vi "MeasurementServer_Start.vi"(7 "error in (no error)":errorcluster, 8 "Server Key File (.key)":path, 9 "Server Certificate File (.crt)":path, 10 "Server Address":string) -> (0 "error out":errorcluster, 2 "Event Registration Refnum":refnum<event-registration>, 3 "Server Information":T2)   [LabVIEW 2019, in "labview-grpc-measurement-server.lvlib"]
uses:
  labview-grpc-measurement-server.lvlib
  MeasurementServer_InvokeEventData.ctl
  MeasurementServer_gRPCid.ctl
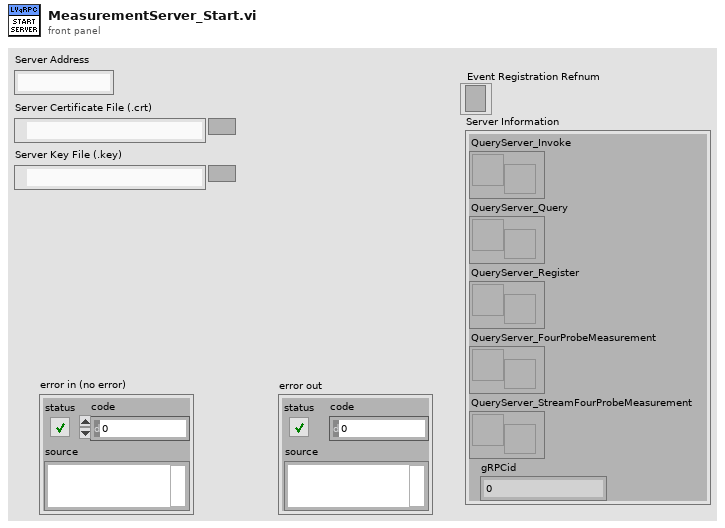
[diagram p1: front panel]
types:
  T1 = typedef "labview-grpc-measurement-server.lvlib/MeasurementServer_gRPCid.ctl" = u64
  T2 = cluster{"QueryServer_Invoke":refnum<user-event>, "QueryServer_Query":refnum<user-event>, "QueryServer_Register":refnum<user-event>, "QueryServer_FourProbeMeasurement":refnum<user-event>, "QueryServer_StreamFourProbeMeasurement":refnum<user-event>, "gRPCid":T1}
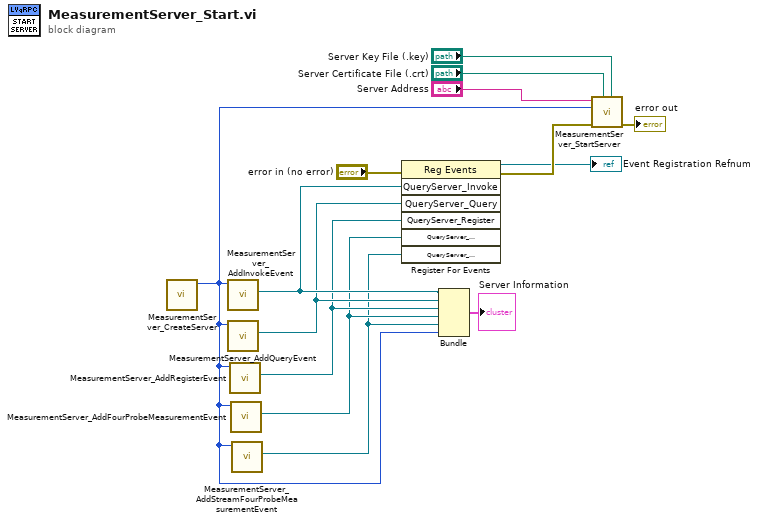
[diagram p0: block diagram]
diagram:
  n1 = call "MeasurementServer_CreateServer.vi"() -> ("gRPCid"=w4:T1)  [unwired: 11 in]
  n2 = call "MeasurementServer_AddInvokeEvent.vi"("gRPCid in"=w4) -> ("QueryServer_Invoke"=w9:refnum<user-event>)  [unwired: 9 in, 1 out]
  n3 = call "MeasurementServer_AddQueryEvent.vi"("gRPCid in"=w4) -> ("QueryServer_Query"=w8:refnum<user-event>)  [unwired: 9 in, 1 out]
  n4 = call "MeasurementServer_AddRegisterEvent.vi"("gRPCid in"=w4) -> ("QueryServer_Register"=w7:refnum<user-event>)  [unwired: 9 in, 1 out]
  n5 = call "MeasurementServer_AddFourProbeMeasurementEvent.vi"("gRPCid in"=w4) -> ("QueryServer_FourProbeMeasurement"=w6:refnum<user-event>)  [unwired: 9 in, 1 out]
  n6 = call "MeasurementServer_AddStreamFourProbeMeasurementEvent.vi"("gRPCid in"=w4) -> ("QueryServer_StreamFourProbeMeasurement"=w5:refnum<user-event>)  [unwired: 9 in, 1 out]
  n7 = register-events(error in="error in (no error)", w9, w8, w7, w6, w5) -> (reference out=→"Event Registration Refnum":refnum<event-registration>, error out=w10:errorcluster)  [unwired: 1 in]
  n8 = Bundle("QueryServer_Invoke"=w9, "QueryServer_Query"=w8, "QueryServer_Register"=w7, "QueryServer_FourProbeMeasurement"=w6, "QueryServer_StreamFourProbeMeasurement"=w5, "gRPCid"=w4) -> (→"Server Information":T2)  [unwired: 1 in]
  n9 = call "MeasurementServer_StartServer.vi"("Server Key File (.key)"="Server Key File (.key)", "Server Certificate File (.crt)"="Server Certificate File (.crt)", "error in (no error)"=w10, "gRPCid"=w4, "Server Address"="Server Address") -> ("error out"=→"error out":errorcluster)  [unwired: 6 in]
